vi "RT Main no FPGA.vi"() -> ()   [LabVIEW 2017]
doc: "The myRIO Custom FPGA Project template acquires button data from the onboard button and displays the button value on a Boolean indicator. The SYS.RDY indicator shows the FPGA status."
uses:
  Controls/Image Size.ctl
  <vilib>/userdefined/High Color/IMAQdx.ctl
  <vilib>/vision/driver/NI_Vision_Acquisition_Software.lvlib
  <vilib>/vision/NI_Vision_Development_Module.lvlib
panel:
  out "FPS":dbl format="%#_6f"
  out "Loop Rate":u32
  out "error out":errorcluster
  in  "Stop":bool
  # "Overview: The myRIO Custom FPGA Project template acquires button data from the onboard button and displays the button value on a Boolean indicator. The SYS.RDY indicator shows the FPGA status.\nRequirements: \n1. LabVIEW FPGA Module.\n2. Xilinx Compilation Tools.\nInstructions:\n1. Check the myRIO target IP address in the project and make sure the target IP address is correct. \n2. Run this VI.\n3. Press the button on the myRIO device."
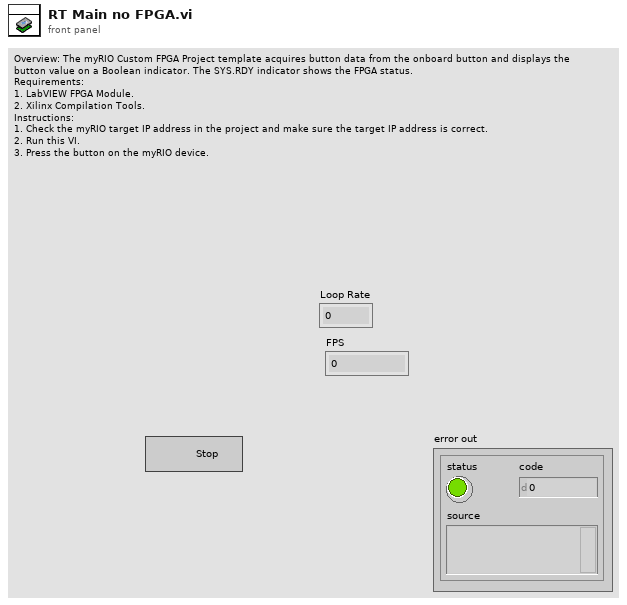
[diagram p1: front panel]
types:
  T1 = typedef "IMAQdx.ctl" = refnum<k21>
  T2 = typedef "Image Size.ctl" = cluster{"Rows (X)":u16, "Colums (Y)":u16}
  T3 = typedef "Image Type" = u32
  T4 = typedef "IMAQ Image.ctl" = refnum<image>
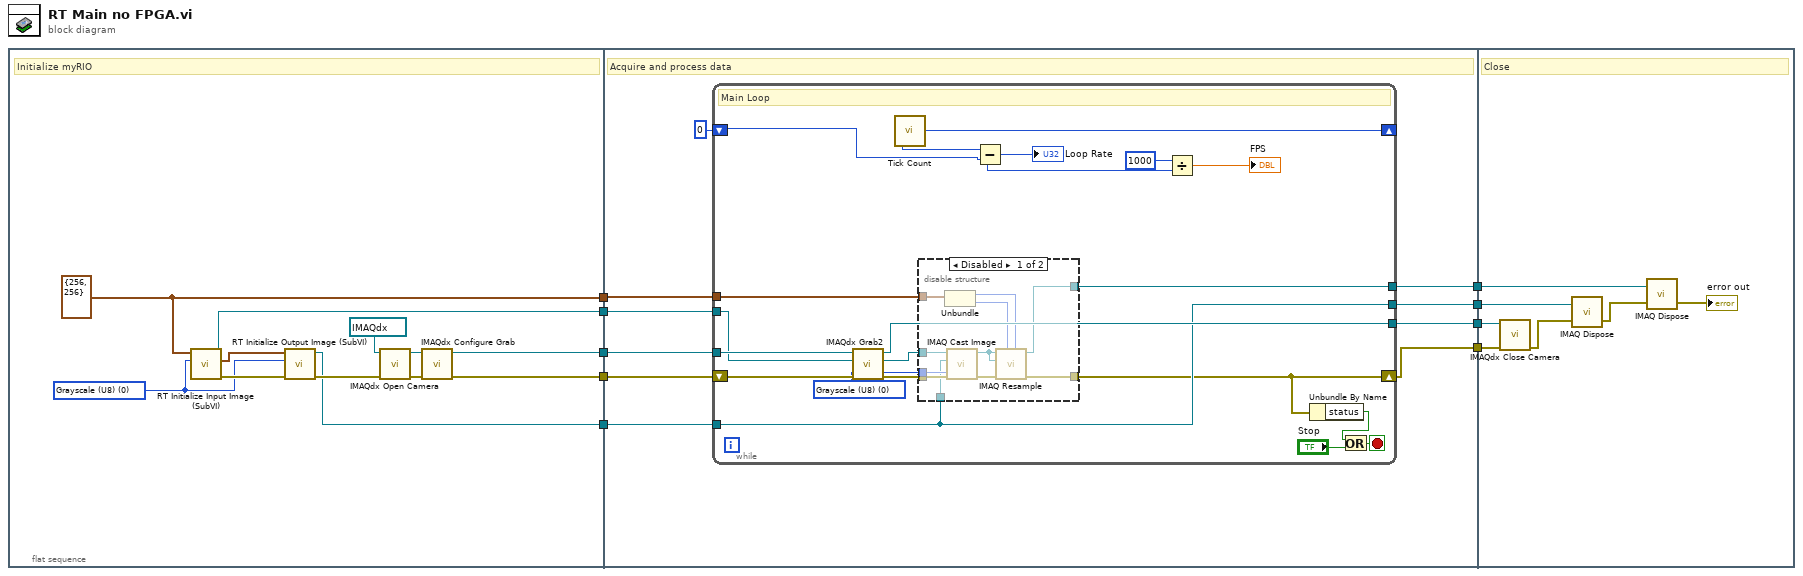
[diagram p0: block diagram]
diagram:
  n1 = flat-sequence {
    tunnel: [w11] -> w9
    tunnel: [w14] -> w7
    tunnel: [w18] -> w6
    tunnel: [w12] -> w5
    tunnel: [w10] -> w4
    tunnel: w9 -> [w31]
    tunnel: [w30] -> w8
    tunnel: w7 -> [w28]
    tunnel: w6 -> [w27]
    tunnel: w5 -> [w26]
    tunnel: w4 -> [w25]
    tunnel: [w24] -> w3
    tunnel: [w23] -> w2
    tunnel: [w22] -> w1
    tunnel: w8 -> [w69]
    tunnel: w3 -> [w70]
    tunnel: w2 -> [w67]
    tunnel: w1 -> [w68]
    frame #0 {
      w12 = T2 {"Rows (X)"=256, "Colums (Y)"=256} ("Image Size")
      w15 = T3 0 items=["Grayscale (U8)", "Grayscale (I16)", "Grayscale (SGL)", "Complex (CSG)", "RGB (U32)", "HSL (U32)", "RGB (U64)", "Grayscale (U16)"] ("Image Type")
      # "Initialize myRIO"
      n2 = call "RT Initialize Input Image (SubVI).vi"("Image Type"=w15, "Image Size In"=w12) -> ("error out"=w17:errorcluster, "Input Image Size Out"=w13:T2, "Input Image Out"=w10:T4)  [unwired: 7 in]
      n3 = call "RT Initialize Output Image (SubVI).vi"("error in (no error)"=w17, "Image Type"=w15, "Image Size In"=w13) -> ("error out"=w16:errorcluster, "Output Image Out"=w14:T4)  [unwired: 7 in]
      n4 = call <vilib>:"IMAQdx Open Camera.vi"("error in"=w16, "Session In"=T1 "cam0") -> ("error out"=w20:errorcluster, "Session Out"=w19:T1)  [unwired: 8 in]
      n5 = call <vilib>:"IMAQdx Configure Grab.vi"("error in"=w20, "Session In"=w19) -> ("error out"=w11:errorcluster, "Session Out"=w18:T1)  [unwired: 8 in]
    }
    frame #1 {
      # "Acquire and process data"
      n6 = while {
        shift-right: [w33] -> w30
        shift-left: w31 -> [w42]
        shift-right: [w48] -> _
        shift-left: u32 0 ("Tick Count(mSec)") -> [w47]
        tunnel: w28 -> [w36]
        tunnel: w26 -> [w34]
        tunnel: w27 -> [w43]
        tunnel: w25 -> [w39]
        tunnel: [w37] -> w24
        tunnel: [w32] -> w23
        tunnel: [w36] -> w22
        stop <- w49 stop-if-true
        w40 = T3 0 items=["Grayscale (U8)", "Grayscale (I16)", "Grayscale (SGL)", "Complex (CSG)", "RGB (U32)", "HSL (U32)", "RGB (U64)", "Grayscale (U16)"] ("Image Type")
        # "Main Loop"
        n7 = call <vilib>:"IMAQdx Grab2.vi"("error in"=w42, "Image In"=w39, "Session In"=w43) -> ("error out"=w41:errorcluster, "Image Out"=w38:T4, "Session Out"=w37:T1)  [unwired: 5 in, 1 out]
        n8 = call "Tick Count"() -> ("Tick Count(mSec)"=w48:u32)
        n9 = disable-structure shown="Disabled" {
          disable-tunnel: w41 -> [w61 w63]
          disable-tunnel: w40 -> [w60 _]
          disable-tunnel: w38 -> [w59 w62]
          disable-tunnel: w36 -> [w58 _]
          disable-tunnel: [w56 w62] -> w32
          disable-tunnel: w34 -> [w54 _]
          disable-tunnel: [w51 w63] -> w33
          frame Disabled {
            n10 = Unbundle(w54) -> ("Rows (X)"=w52:u16, "Colums (Y)"=w53:u16)
            n11 = call "IMAQ Cast Image"("Image Type"=w60, "error in (no error)"=w61, "Image Dst"=w58, "Image Src"=w59) -> ("error out"=w57:errorcluster, "Image Dst Out"=w55:T4)  [unwired: 6 in]
            n12 = call "IMAQ Resample"("X Resolution"=w52, "Y Resolution"=w53, "error in (no error)"=w57, "Image Dst"=w55, "Image Src"=w55) -> ("error out"=w51:errorcluster, "Image Dst Out"=w56:T4)  [unwired: 5 in]
          }
          frame Enabled {
          }
        }
        n13 = Subtract(x=w48, y=w47) -> (x-y=w46:u32)
        "Loop Rate" <- w46
        n14 = Divide(x=u32 1000, y=w46) -> (x/y=→"FPS":dbl)
        n15 = Unbundle By Name(w33) -> ("status"=w35:bool)
        n16 = Or(x=w35, y="Stop") -> (x .or. y?=w49:bool)
      }
    }
    frame #2 {
      # "Close"
      n17 = call <vilib>:"IMAQdx Close Camera.vi"("error in"=w69, "Session In"=w70) -> ("error out"=w66:errorcluster)  [unwired: 9 in]
      n18 = call "IMAQ Dispose"("Image"=w68, "error in (no error)"=w66) -> ("error out"=w65:errorcluster)  [unwired: 4 in]
      n19 = call "IMAQ Dispose"("Image"=w67, "error in (no error)"=w65) -> ("error out"=→"error out":errorcluster)  [unwired: 4 in]
    }
  }
